vi "Write String Delimiter.vi"(8 "error in (no error)":errorcluster, 10 "String Delimiter":string=",", 11 "Abs_Boolean_1D in":refnum<class "Abs_Boolean_1D.lvclass">) -> (0 "error out":errorcluster, 3 "Abs_Boolean_1D out":refnum<class "Abs_Boolean_1D.lvclass">)   [LabVIEW 2021, in "Abs_Boolean_1D.lvclass"]
uses:
  Abs_Boolean_1D.lvclass
  Abs_Boolean_1D.lvclass/Abs_Boolean_1D.ctl
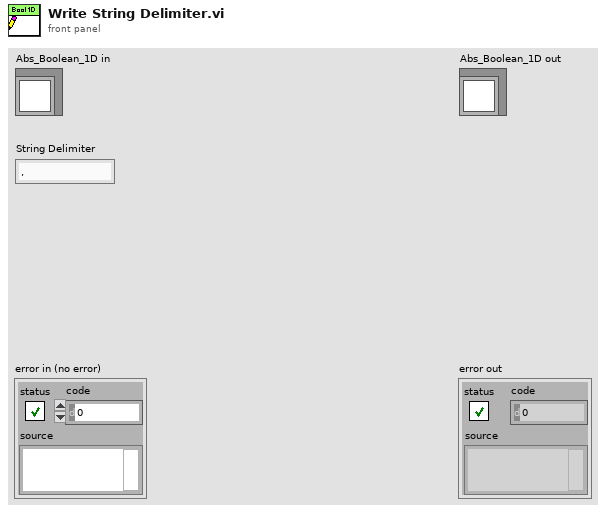
[diagram p1: front panel]
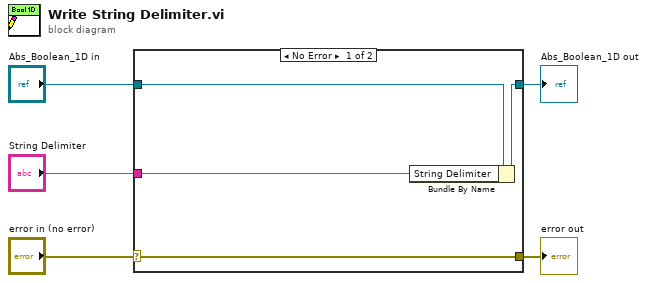
[diagram p0: block diagram]
diagram:
  n1 = case shown="No Error" "error in (no error)" {
    selector: "error in (no error)" -> [w9 w10]
    tunnel: [w9 w10] -> w4
    tunnel: [w7 w11] -> w2
    tunnel: "Abs_Boolean_1D in" -> [w8 w11]
    tunnel: "String Delimiter" -> [w6 _]
    frame No Error {
      n2 = Bundle By Name(cluster=w8, "String Delimiter"=w6) -> (w7:refnum<class "Abs_Boolean_1D.lvclass">)
    }
    frame Error {
    }
  }
  "error out" <- w4
  "Abs_Boolean_1D out" <- w2
